vi "arduino serial write P.vi"(8 "error in":errorcluster, 9 "DAC value (0-1024)":string, 10 "DAC output":string(combo), 11 "Pressure Box COM":refnum<visa-resource-name>) -> (0 "error out":errorcluster, 3 "Pressure Box COM out":refnum<visa-resource-name>)   [LabVIEW 2019]
uses:
  <vilib>/Instr/_visa.llb/VISA Flush IO Buffer Mask.ctl
panel:
  out "Response":string
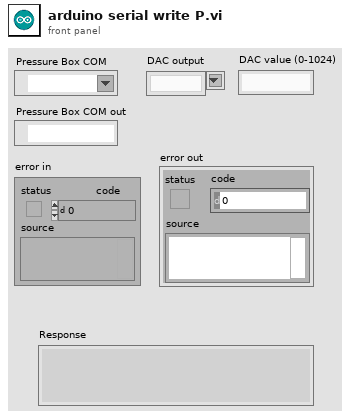
[diagram p1: front panel]
types:
  T1 = typedef "VISA Flush IO Buffer Mask.ctl" = u16
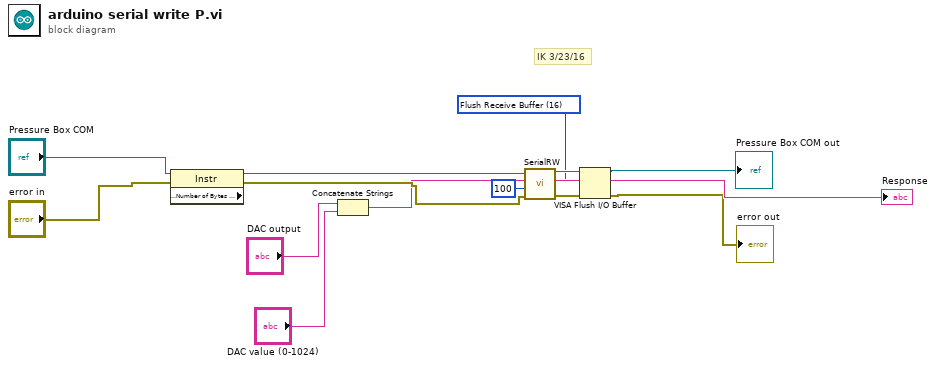
[diagram p0: block diagram]
diagram:
  w1 = T1 16 items=["Flush Receive Buffer"=16, "Write Transmit Buffer to Device"=32, "Flush Receive Buffer (No I/O)"=64, "Flush Transmit Buffer"=128] ("Mask")
  # "IK 3/23/16"
  n1 = property class="Instr" props=["Serial Settings:Number of Bytes at Serial Port"](reference="Pressure Box COM", error in="error in") -> (reference out=w12:refnum<visa-resource-name>, error out=w11:errorcluster)  [unwired: 1 out]
  n2 = Concatenate Strings("DAC output", "DAC value (0-1024)") -> (w10:string)
  n3 = call "SerialRW.vi"("error in (no error)"=w11, "Delay (ms)"=u32 100, "Command"=w10, "VISA handle"=w12) -> ("error out"=w2:errorcluster, "Response"=→"Response":string, "Dup. VISA handle"=w5:refnum<visa-resource-name>)  [unwired: 2 in, 1 out]
  n4 = VISA Flush I/O Buffer(VISA resource name=w5, mask (16)=w1, error in (no error)=w2) -> (VISA resource name out=→"Pressure Box COM out":refnum<visa-resource-name>, error out=→"error out":errorcluster)
